vi "Get_Set_Satellites.vi"(6 "Get/Set":T2, 8 "Status/Errors in":refnum<vi>, 9 "Satellites in":refnum<vi>, 11 "Satellites in":T1) -> (0 "Status/Errors out":refnum<vi>, 1 "Satellites out":refnum<vi>, 3 "Satellites out":T1)   [LabVIEW 2010]
uses:
  Controls/Get_Set_Statistics_Options2.ctl
  Controls/Tabpage_Satellites.ctl
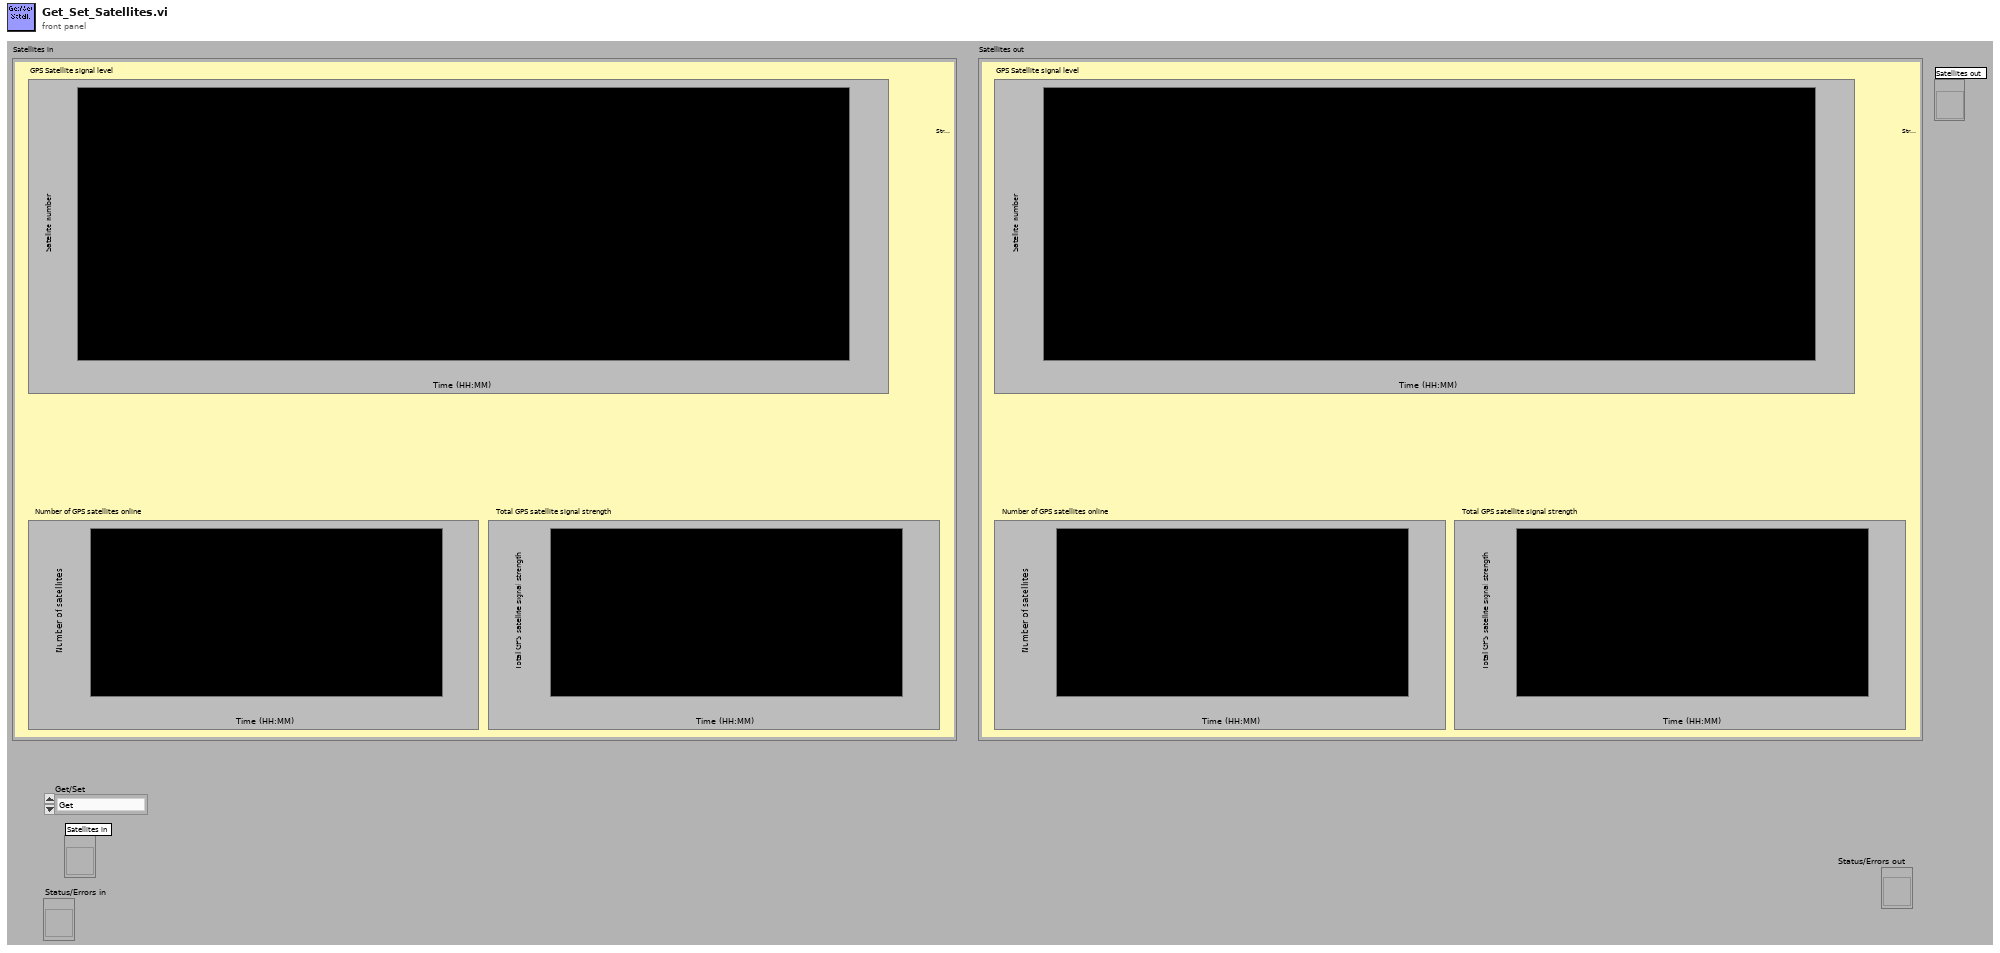
[diagram p1: front panel]
types:
  T1 = typedef "Tabpage_Satellites.ctl" = cluster{"Satellites_online":dbl[], "Satellite_signal":dbl[][], "Total_signal_strength":dbl[], "First time?":bool}
  T2 = typedef "Get_Set_Statistics_Options2.ctl" = enum16{"Get", "Set"}
  T3 = cluster{"Satellites_online":dbl[], "Satellite_signal":dbl[][], "Total_signal_strength":dbl[], "First time?":bool}
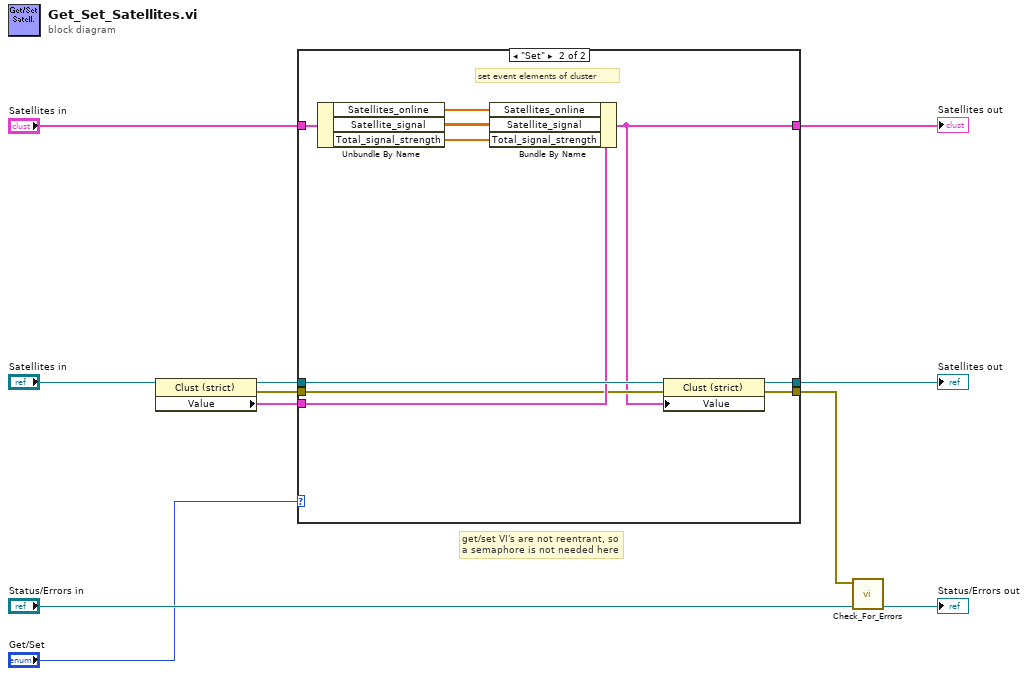
[diagram p0: block diagram]
diagram:
  # "get/set VI's are not reentrant, so\na semaphore is not needed here"
  n1 = property class="Clust (strict)"(reference="Satellites in") -> (reference out=w8:refnum<vi>, error out=w7:errorcluster, "Value"=w6:T3)  [unwired: 1 in]
  n2 = case shown="\"Set\"" "Get/Set" {
    tunnel: "Satellites in" -> [_ w19]
    tunnel: w8 -> [w14 w24]
    tunnel: [w14 w22] -> w1
    tunnel: [w13 w23] -> w10
    tunnel: [w12 w18] -> w4
    tunnel: w6 -> [w12 w21]
    tunnel: w7 -> [w13 w20]
    frame "Get" {
      # "get cluster"
    }
    frame "Set" {
      # "set event elements of cluster"
      n3 = Unbundle By Name(w19) -> ("Satellites_online"=w17:dbl[], "Satellite_signal"=w16:dbl[][], "Total_signal_strength"=w15:dbl[])
      n4 = Bundle By Name(cluster=w21, "Satellites_online"=w17, "Satellite_signal"=w16, "Total_signal_strength"=w15) -> (w18:T3)
      n5 = property class="Clust (strict)"(reference=w24, error in=w20, "Value"=w18) -> (reference out=w22:refnum<vi>, error out=w23:errorcluster)
    }
  }
  "Satellites out" <- w4
  "Satellites out" <- w1
  n6 = call "Check_For_Errors.vi"("Status/Errors in"="Status/Errors in", "error in"=w10) -> ("Status/Errors out"=→"Status/Errors out":refnum<vi>)  [unwired: 9 out]
